vi "Message List FGV.vi"(6 "Action (Get)":T1, 8 "error in (no error)":errorcluster, 11 "Message Object":refnum<class>) -> (0 "error out":errorcluster, 3 "Messages":string[](array[string]))   [LabVIEW 2027]
uses:
  Message List Action.ctl
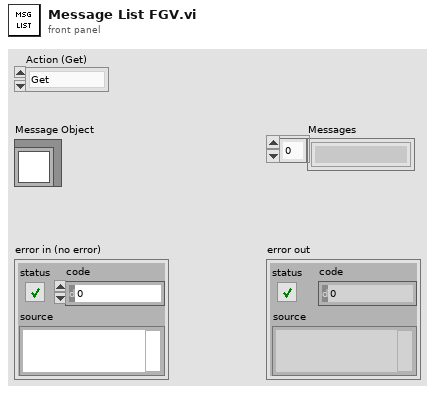
[diagram p1: front panel]
types:
  T1 = typedef "Message List Action.ctl" = enum16{"Get", "Add", "Reset"}
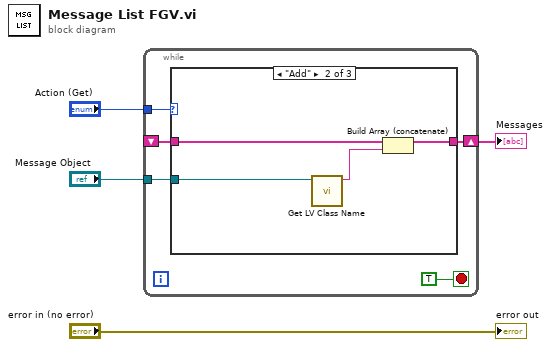
[diagram p0: block diagram]
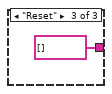
[diagram p3: hidden frame]
diagram:
  n1 = while {
    tunnel: "Action (Get)" -> [w8]
    shift-right: [w7] -> w2
    shift-left: _ -> [w6]
    tunnel: "Message Object" -> [w5]
    stop <- TRUE stop-if-true
    n2 = case shown="\"Add\"" w8 {
      tunnel: [w10 w13 string[] []] -> w7
      tunnel: w6 -> [w10 w14 _]
      tunnel: w5 -> [_ w11 _]
      frame "Get", Default {
      }
      frame "Add" {
        n3 = call <vilib>:"Get LV Class Name.vi"("object"=w11) -> ("class name"=w12:string)  [unwired: 9 in, 1 out]
        n4 = Build Array (concatenate)(w14, w12) -> (w13:string[])
      }
      frame "Reset" {
      }
    }
  }
  "Messages" <- w2
  "error out" <- "error in (no error)"
